vi "1.vi"() -> ()   [LabVIEW 2017]
panel:
  out "元素 4":dbl
  out "元素 3":dbl
  out "元素 2":dbl
  out "元素":dbl
  out "数组":dbl[](array[numeric])
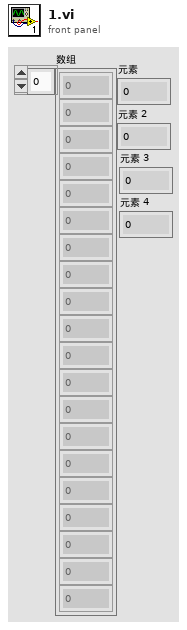
[diagram p1: front panel]
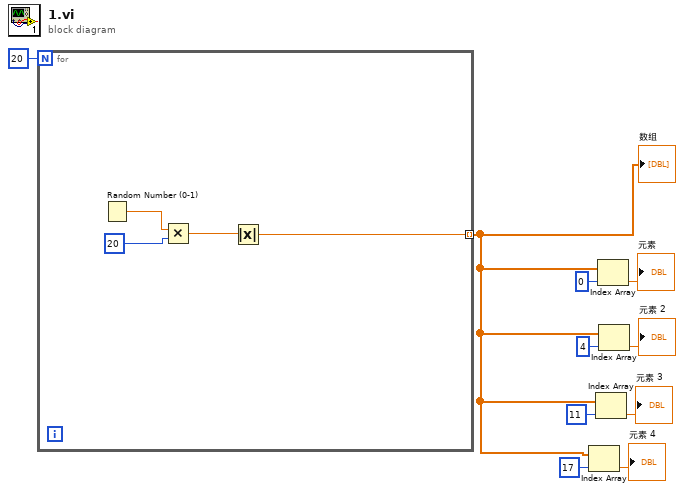
[diagram p0: block diagram]
diagram:
  n1 = for {
    N: 20 -> [_]
    tunnel: [w11] -> w5 mode=indexing
    n2 = Random Number (0-1)() -> (number: 0 to 1=w14:dbl)
    n3 = Multiply(x=w14, y=20) -> (x*y=w12:dbl)
    n4 = Absolute Value(x=w12) -> (abs(x)=w11:dbl)
  }
  "数组" <- w5
  n5 = Index Array(array=w5, index=17 ("索引")) -> (element=→"元素 4":dbl)
  n6 = Index Array(array=w5, index=11 ("索引")) -> (element=→"元素 3":dbl)
  n7 = Index Array(array=w5, index=0 ("索引")) -> (element=→"元素":dbl)
  n8 = Index Array(array=w5, index=4 ("索引")) -> (element=→"元素 2":dbl)
